vi "write_udc_float.vi"(1 "Value":dbl, 2 "Hex Address":u16 format="%x") -> ()   [LabVIEW 2011]
uses:
  <vilib>/NI Modbus.llb/MB Ethernet Master Query Write Multiple Registers (poly).vi
panel:
  out "Error Out":errorcluster
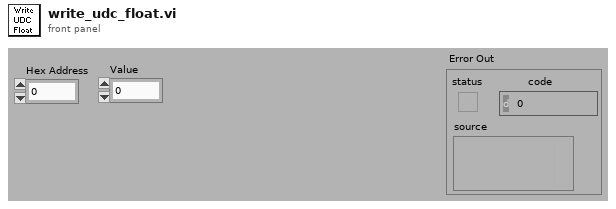
[diagram p1: front panel]
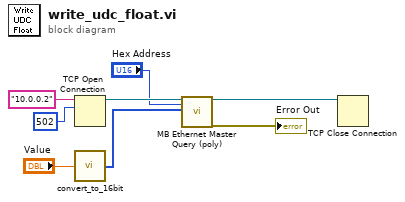
[diagram p0: block diagram]
diagram:
  n1 = TCP Open Connection(address="10.0.0.2", remote port or service name=u16 502) -> (connection ID=w6:refnum<k5>)  [unwired: 1 in, 3 out]
  n2 = call "convert_to_16bit.vi"("Floating point"="Value") -> ("Output Array"=w3:u16[])
  n3 = call-poly <vilib>:"MB Ethernet Master Query (poly).vi"("TCP Connection Refnum in"=w6, "Starting Address"="Hex Address", "Registers"=w3) -> ("TCP Connection Refnum (dup)"=w5:refnum<k5>, "error out"=→"Error Out":errorcluster)  [unwired: 3 in, 12 out]
  n4 = TCP Close Connection(connection ID=w5) -> ()  [unwired: 1 in, 3 out]
